vi "Create.vi"(8 "error in (no error)":errorcluster, 9 "Resolution":i32, 11 "Reference":refnum<vi>) -> (0 "error out":errorcluster, 1 "To Control":T1, 3 "BigMAQ out":refnum<class "BigMAQ.lvclass">)   [LabVIEW 2019, in "BigMAQ.lvclass"]
uses:
  BigMAQ.lvclass
  <vilib>/vision/Image Controls.llb/IMAQ Image.ctl
  BigMAQ.lvclass/BigMAQ.ctl
  <vilib>/LabVIEW Open Source Project/Unicity/RandomStringGenerator/RandomStringGenerator.lvclass
panel:
  in  "BigMAQ in":refnum<class "BigMAQ.lvclass">
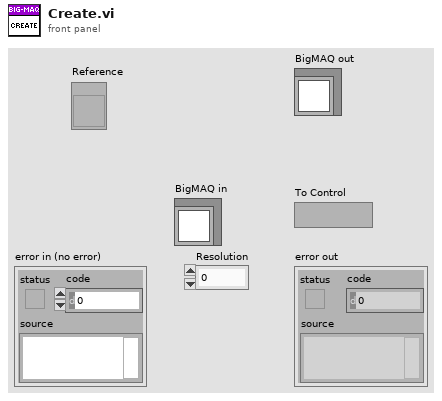
[diagram p1: front panel]
types:
  T1 = typedef "IMAQ Image.ctl" = refnum<image>
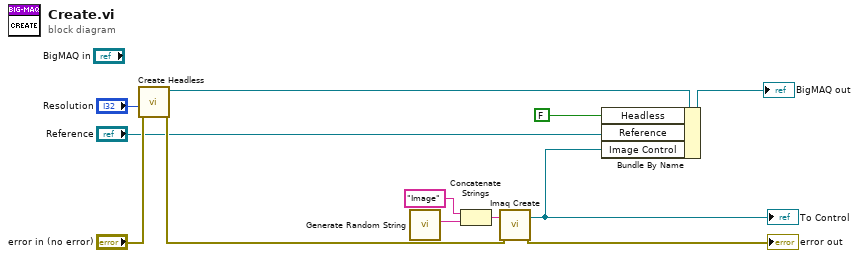
[diagram p0: block diagram]
diagram:
  n1 = call "Create Headless.vi"("error in"="error in (no error)", "Resolution"="Resolution") -> ("error out"=w3:errorcluster, "BigMAQ out"=w10:refnum<class "BigMAQ.lvclass">)  [unwired: 8 in]
  n2 = call <vilib>:"Generate Random String.vi"() -> ("Random String"=w1:string)  [unwired: 11 in]
  n3 = Concatenate Strings("Image" ("Image Name"), w1) -> (w6:string)
  n4 = call "Imaq Create"("Image Name"=w6, "error in (no error)"=w3) -> ("New Image"=w5:T1, "error out"=→"error out":errorcluster)  [unwired: 3 in]
  "To Control" <- w5
  n5 = Bundle By Name(cluster=w10, "Headless"=FALSE, "Reference"="Reference", "Image Control"=w5) -> (→"BigMAQ out":refnum<class "BigMAQ.lvclass">)
